vi "Configurations UI.vi"() -> ()   [LabVIEW 2020, in "Performance Monitor UI.lvlib" / "Configuration.lvlib"]
doc: "Module UI that appears in the DCFG Framework for the Configurations View.\n_____\nBased on DCFG Project Template 1.0.0.21.\n____\nPeloton Config 1.0.0.2\nCopyright (c) 2022, Peloton"
uses:
  Configuration.lvlib
  <vilib>/Delacor/Delacor QMH/Libraries/Cloneable Module Admin_class/Delacor_lib_QMH_Cloneable Module Admin.lvclass
  Configuration--cluster.ctl
  <vilib>/Peloton/Peloton Config/Libraries/DCFG Page/Peloton_DCFG Page.lvlib
panel:
  out "Current Default Configuration":T1
  in  "Random Path":path
  in  "Module Admin":refnum<class "Delacor_lib_QMH_Cloneable Module Admin.lvclass">
  in  "Values in":variant
  in  "Initialized":refnum<notifier>
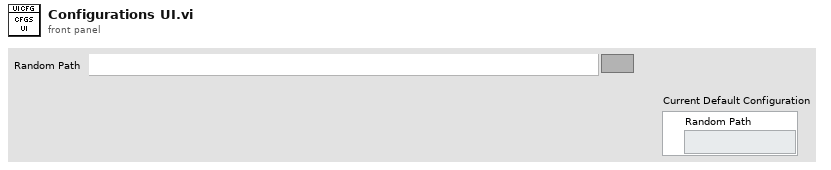
[diagram p1: front panel]
types:
  T1 = typedef "Performance Monitor UI.lvlib/Configuration.lvlib/Configuration--cluster.ctl" = cluster{"Random Path":path}
  T2 = enum32{"Invalid", "Standard", "Closed", "Hidden", "Minimized", "Maximized"}
  T3 = typedef "Rename As Application UI.lvlib/Configuration.lvlib/Configuration--cluster.ctl" = cluster{"Random Path":path}
  T4 = typedef "Peloton_DCFG Page.lvlib/Broadcast Events--cluster.ctl" = cluster{"Module Did Init":refnum<user-event>, "Status Updated":refnum<user-event>, "Error Reported":refnum<user-event>, "Module Did Stop":refnum<user-event>, "Send Data":refnum<user-event>, "Receive Data":refnum<user-event>, "Defaults Set":refnum<user-event>, "Update Module Execution Status":refnum<user-event>, "Unapplied Changes":refnum<user-event>}
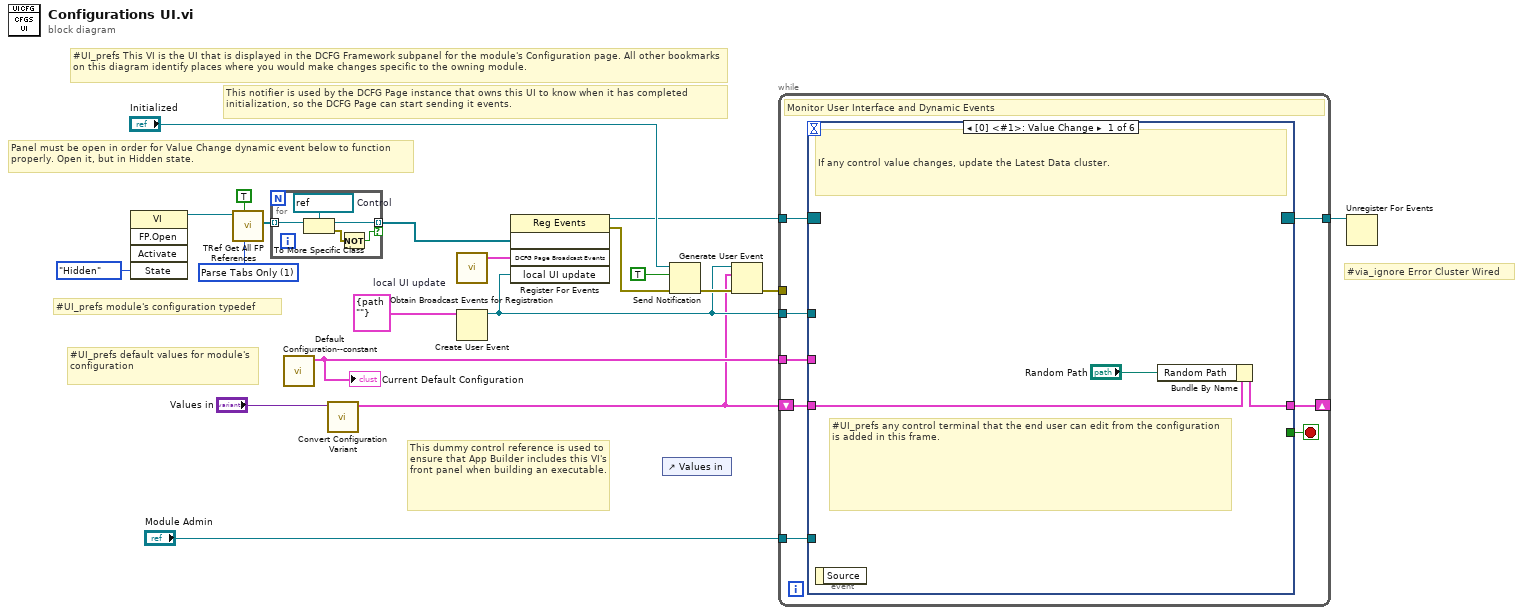
[diagram p0: block diagram]
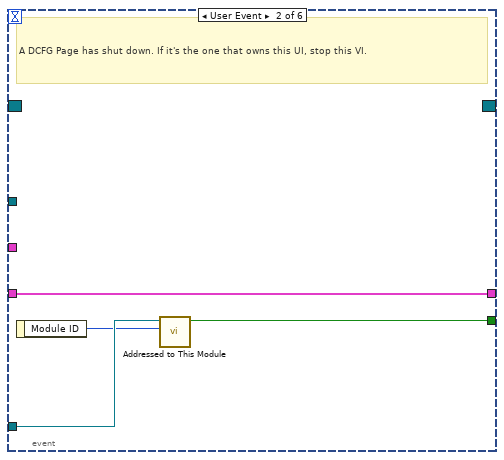
[diagram p2: hidden frame]
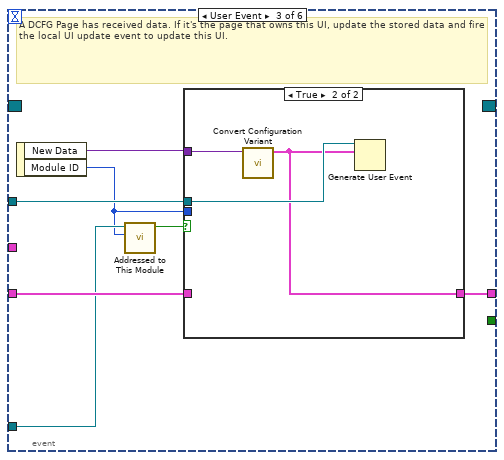
[diagram p3: hidden frame]
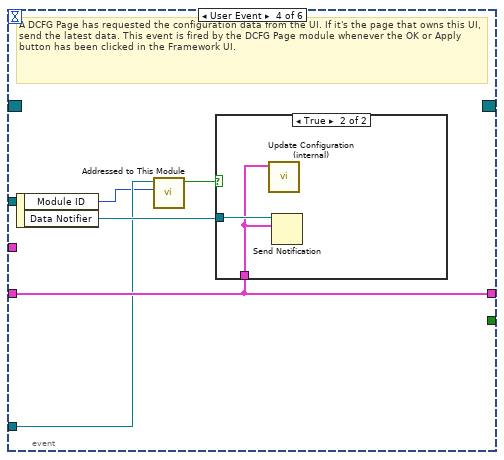
[diagram p5: hidden frame]
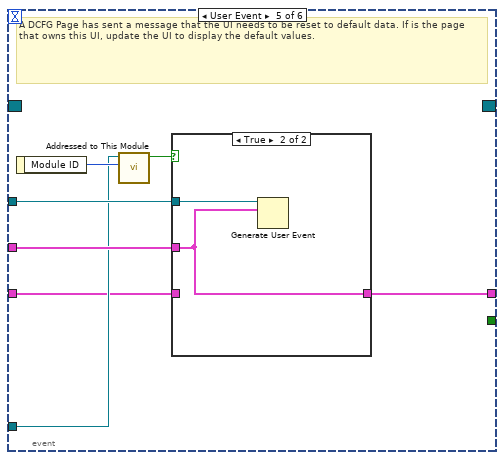
[diagram p7: hidden frame]
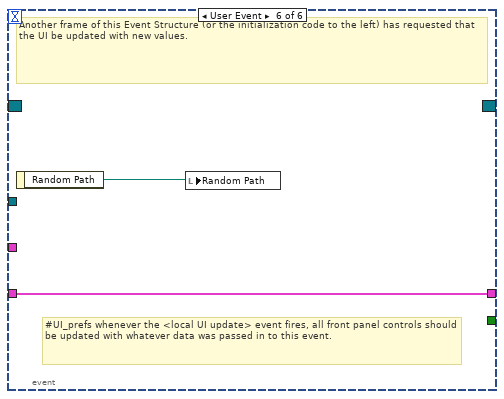
[diagram p9: hidden frame]
diagram:
  w4 = u16 1 items=["Parse All", "Parse Tabs Only"] ("Parsing Rule")
  w11 = T1 {"Random Path"=path ""}  # local UI update
  # "#via_ignore Error Cluster Wired"
  # "This dummy control reference is used to ensure that App Builder includes this VI's front panel when building an executable."
  # "Panel must be open in order for Value Change dynamic event below to function properly. Open it, but in Hidden state."
  # "This notifier is used by the DCFG Page instance that owns this UI to know when it has completed initialization, so the DCFG Page can start sending it events."
  # "#UI_prefs module's configuration typedef"
  # "#UI_prefs default values for module's configuration"
  # "#UI_prefs This VI is the UI that is displayed in the DCFG Framework subpanel for the module's Configuration page. All other bookmarks on this diagram identify places where you would make changes specific to the owning module."
  n1 = invoke class="VI" method="FP.Open"("State"=T2."Hidden") -> (reference out=w2:refnum<vi>)  [unwired: 4 in, 4 out]
  n2 = call <vilib>:"TRef Get All FP References.vi"("Parsing Rule"=w4, "Ignore Decorations?"=TRUE, "VI Refnum"=w2) -> ("All FP Objects"=w3:refnum<vi>[])  [unwired: 4 in, 4 out]
  n3 = for {
    tunnel: w3 -> [w25] mode=indexing
    tunnel: [w24] -> w1 mode=indexing if=w21
    w23 = refnum<vi> refnum  # Control
    n4 = To More Specific Class(target class=w23, reference=w25) -> (specific class reference=w24:refnum<vi>, error out=w22:errorcluster)  [unwired: 1 in]
    n5 = Not(x=w22) -> (.not. x?=w21:bool)
  }
  n6 = call "Default Configuration--constant.vi"() -> ("Default Configuration"=w8:T3)  [unwired: 11 in]
  "Current Default Configuration" <- w8
  n7 = call "Convert Configuration Variant.vi"("Current Configuration"="Values in") -> ("Configuration"=w6:T1)  [unwired: 8 in, 2 out]
  n8 = call <vilib>:"Obtain Broadcast Events for Registration.vi"() -> ("DCFG Page Broadcast Events"=w19:T4)  [unwired: 9 in, 2 out]
  n9 = Create User Event(user event datatype=w11) -> (user event=w9:refnum<user-event>)  [unwired: 1 in, 1 out]
  n10 = register-events(w1, w19, w9) -> (reference out=w15:refnum<event-registration>, error out=w13:errorcluster)  [unwired: 2 in]
  n11 = control-ref of="Values in"() -> ()  [unwired: 1 out]
  n12 = Send Notification(notification=TRUE, notifier="Initialized", error in (no error)=w13) -> (error out=w16:errorcluster)  [unwired: 1 out]
  n13 = Generate User Event(user event=w9, event data cluster=w6, error in=w16) -> (error out=w10:errorcluster)  [unwired: 1 in, 1 out]
  n14 = while {
    tunnel: w10 -> [_]
    tunnel: w15 -> [w33]
    tunnel: [w32] -> w14
    shift-right: [w28] -> _
    shift-left: w6 -> [w31]
    tunnel: "Module Admin" -> [w29]
    tunnel: w8 -> [w27]
    tunnel: w9 -> [w26]
    stop <- w30 stop-if-true
    # "Monitor User Interface and Dynamic Events"
    n15 = event shown="[0] <#1>: Value Change" {
      selector: w33 -> [_ _ _ _ _ _]
      dyn-events: [_ _ _ _ _ _] -> w32
      timeout: _ -> [_ _ _ _ _ _]
      tunnel: w31 -> [w36 w40 w47 w55 w60 w70]
      tunnel: [w35 w40 w46 w55 w59 w70] -> w28
      tunnel: [_ w37 _ _ _ _] -> w30
      tunnel: w29 -> [_ w39 w42 w54 w62 _]
      tunnel: w27 -> [_ _ _ _ w65 _]
      tunnel: w26 -> [_ _ w44 _ w64 _]
      event Value Change {
        # "#UI_prefs any control terminal that the end user can edit from the configuration is added in this frame."
        # "If any control value changes, update the Latest Data cluster."
        n16 = event-data() -> ()  [unwired: 1 in, 1 out]
        n17 = Bundle By Name(cluster=w36, "Random Path"="Random Path") -> (w35:T1)
      }
      event User Event {
        # "A DCFG Page has shut down. If it's the one that owns this UI, stop this VI."
        n18 = event-data() -> ("Module ID"=w38:i32)  [unwired: 1 in]
        n19 = call <vilib>:"Addressed to This Module.vi"("Module ID from Argument"=w38, "Module Admin"=w39) -> ("Addressed to this instance?"=w37:bool)  [unwired: 8 in, 1 out]
      }
      event User Event {
        # "A DCFG Page has received data. If it's the page that owns this UI, update the stored data and fire the local UI update event to update this UI."
        n20 = event-data() -> ("New Data"=w45:variant, "Module ID"=w41:i32)  [unwired: 1 in]
        n21 = call <vilib>:"Addressed to This Module.vi"("Module ID from Argument"=w41, "Module Admin"=w42) -> ("Addressed to this instance?"=w43:bool)  [unwired: 8 in, 1 out]
        n22 = case shown="True" w43 {
          tunnel: w47 -> [w48 _]
          tunnel: [w48 w49] -> w46
          tunnel: w45 -> [_ w50]
          tunnel: w44 -> [_ w51]
          tunnel: w41 -> [_ _]
          frame False {
          }
          frame True {
            n23 = call "Convert Configuration Variant.vi"("Current Configuration"=w50) -> ("Configuration"=w49:T1)  [unwired: 8 in, 2 out]
            n24 = Generate User Event(user event=w51, event data cluster=w49) -> ()  [unwired: 2 in, 2 out]
          }
        }
      }
      event User Event {
        # "A DCFG Page has requested the configuration data from the UI. If it's the page that owns this UI, send the latest data. This event is fired by the DCFG Page module whenever the OK or Apply button has been clicked in the Framework UI."
        n25 = event-data() -> ("Module ID"=w52:i32, "Data Notifier"=w56:refnum<notifier>)  [unwired: 1 in]
        n26 = call <vilib>:"Addressed to This Module.vi"("Module ID from Argument"=w52, "Module Admin"=w54) -> ("Addressed to this instance?"=w53:bool)  [unwired: 8 in, 1 out]
        n27 = case shown="True" w53 {
          tunnel: w56 -> [_ w58]
          tunnel: w55 -> [_ w57]
          frame False {
          }
          frame True {
            n28 = call "Update Configuration (internal).vi"("configuration"=w57) -> ()  [unwired: 11 in]
            n29 = Send Notification(notification=w57, notifier=w58) -> ()  [unwired: 1 in, 2 out]
          }
        }
      }
      event User Event {
        # "A DCFG Page has sent a message that the UI needs to be reset to default data. If is the page that owns this UI, update the UI to display the default values."
        n30 = event-data() -> ("Module ID"=w63:i32)  [unwired: 1 in]
        n31 = call <vilib>:"Addressed to This Module.vi"("Module ID from Argument"=w63, "Module Admin"=w62) -> ("Addressed to this instance?"=w61:bool)  [unwired: 8 in, 1 out]
        n32 = case shown="True" w61 {
          tunnel: w65 -> [_ w67]
          tunnel: w64 -> [_ w68]
          tunnel: w60 -> [w66 _]
          tunnel: [w66 w67] -> w59
          frame False {
          }
          frame True {
            n33 = Generate User Event(user event=w68, event data cluster=w67) -> ()  [unwired: 2 in, 2 out]
          }
        }
      }
      event User Event {
        # "#UI_prefs whenever the <local UI update> event fires, all front panel controls should be updated with whatever data was passed in to this event."
        # "Another frame of this Event Structure (or the initialization code to the left) has requested that the UI be updated with new values."
        n34 = event-data() -> ("Random Path"=w69:path)  [unwired: 1 in]
        n35 = local write "Random Path"(w69) -> ()
      }
    }
  }
  n36 = Unregister For Events(event registration refnum=w14) -> ()  [unwired: 1 in, 1 out]
